vi "DrawPoints.vi"(8 "error in (no error)":errorcluster, 10 "Overlay":T1, 11 "Image":T1) -> (0 "error out":errorcluster, 3 "Image Out":T1)   [LabVIEW 2017, in "ImageAcquisitionLibrary.lvlib"]
uses:
  ImageAcquisitionLibrary.lvlib
  <vilib>/vision/Image Controls.llb/IMAQ Image.ctl
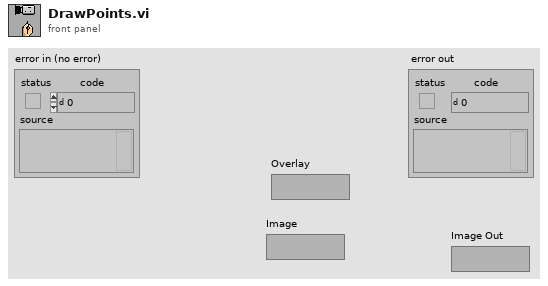
[diagram p1: front panel]
types:
  T1 = typedef "IMAQ Image.ctl" = refnum<image>
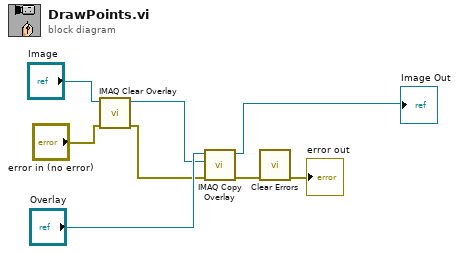
[diagram p0: block diagram]
diagram:
  n1 = call "IMAQ Clear Overlay"("error in (no error)"="error in (no error)", "Image"="Image") -> ("error out"=w1:errorcluster, "Image Out"=w6:T1)  [unwired: 8 in]
  n2 = call "IMAQ Copy Overlay"("error in (no error)"=w1, "Image Dst"=w6, "Image Src"="Overlay") -> ("error out"=w3:errorcluster, "Image Dst Out"=→"Image Out":T1)  [unwired: 7 in]
  n3 = call <vilib>:"Clear Errors.vi"("error in (no error)"=w3) -> ("error out"=→"error out":errorcluster)  [unwired: 5 in, 1 out]
